vi "get_sgl.vi"   [LabVIEW 2012]
uses:
  <vilib>/addons/internet/NI_InternetTK_Core_VIs.lvlib
types:
  T1 = enum16{"(default)", "monospaced", "italic", "bold", "underlined", "strike-through", "big", "small", "superscript", "subscript"}
  T2 = typedef "CGI Connection Info.ctl" = cluster{"name":string, "type":T3, "session":T4}
  T3 = typedef "CGI Request Type.ctl" = enum16{"cgi", ".spool first", ".spool", ".spool last"}
  T4 = typedef "HTTP Session.ctl" = refnum<k1>
  T5 = typedef "NI_FTP.lvlib/Keyed Array.ctl" = cluster{"keys":string[], "values":string[]}
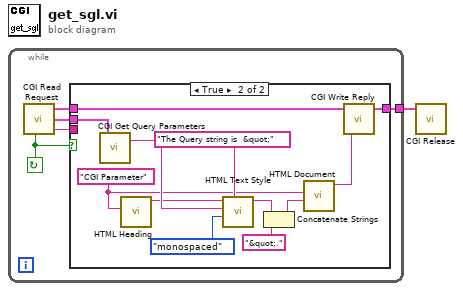
[diagram p0: block diagram]
diagram:
  n1 = while {
    tunnel: [w5] -> w1
    stop <- w4 continue-if-true
    n2 = call <vilib>:"CGI Read Request.vi"() -> ("valid request?"=w4:bool, "cgi connection info"=w6:T2, "env"=w3:T5, "content"=w2:string)  [unwired: 4 in]
    n3 = case shown="True" w4 {
      tunnel: [w7 w19] -> w5
      tunnel: w6 -> [w7 w18]
      tunnel: w3 -> [_ w16]
      tunnel: w2 -> [_ _]
      frame False {
      }
      frame True {
        w11 = "CGI Parameter" ("heading")
        n4 = call <vilib>:"CGI Get Query Parameters.vi"("env"=w16) -> ("query string"=w15:string)  [unwired: 2 out]
        n5 = call <vilib>:"HTML Heading.vi"("heading"=w11) -> ("HTML out"=w14:string)  [unwired: 10 in]
        n6 = call <vilib>:"HTML Text Style.vi"("label"="The Query string is  &quot;", "style (default)"=T1."monospaced", "text"=w15, "HTML in"=w14) -> ("HTML out"=w10:string)  [unwired: 7 in]
        n7 = Concatenate Strings(w10, "&quot;." ("label")) -> (w8:string)
        n8 = call <vilib>:"HTML Document.vi"("document body"=w8, "document title"=w11) -> ("HTML Document"=w17:string)  [unwired: 9 in]
        n9 = call <vilib>:"CGI Write Reply.vi"("content"=w17, "cgi connection info"=w18) -> ("cgi connection info out"=w19:T2)  [unwired: 3 in]
      }
    }
  }
  n10 = call <vilib>:"CGI Release.vi"("cgi connection info"=w1) -> ()  [unwired: 5 in]
